vi "FTW-XML-Query-UpdateFirstElementXML.vi"(0 "Parent Element":refnum<k20>, 5 "XPath Query":string, 7 "New XML Element":string, 11 "error in":errorcluster) -> (4 "Parent Element out":refnum<k20>, 6 "Updated?":bool, 15 "error out":errorcluster)   [LabVIEW 2013]
uses:
  ftw-dataflow/Core/src/Error/FTW-ERR-ThrowError.vi
  <resource>/objmgr/DOMUserDefRef.rc
panel:
  # "Inputs"
  # "Outputs"
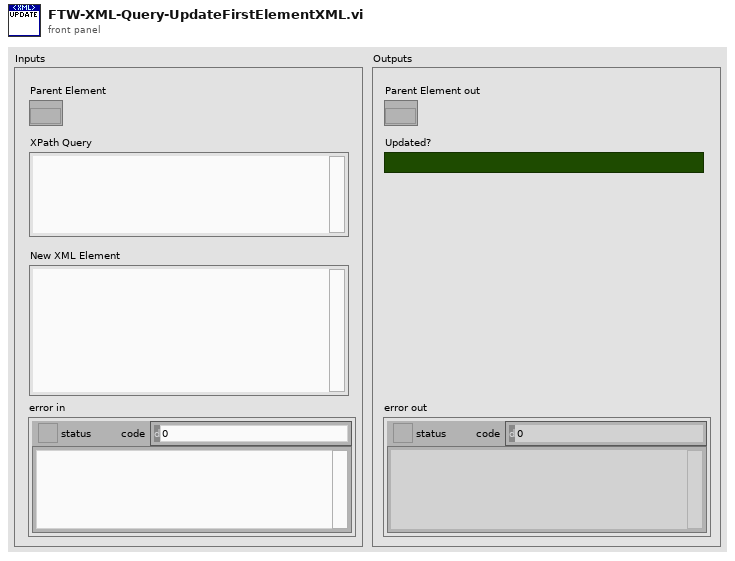
[diagram p1: front panel]
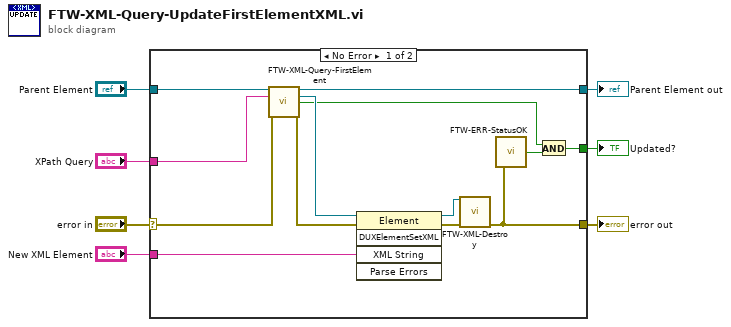
[diagram p0: block diagram]
diagram:
  n1 = case shown="No Error" "error in" {
    selector: "error in" -> [w17 w22]
    tunnel: [w9 w22] -> w7
    tunnel: "Parent Element" -> [w18 w21]
    tunnel: [w16 w21] -> w4
    tunnel: "New XML Element" -> [w20 _]
    tunnel: "XPath Query" -> [w15 _]
    tunnel: [w10 _] -> w1
    frame No Error {
      n2 = call "FTW-XML-Query-FirstElement.vi"("XML Node"=w18, "XPath Query"=w15, "error in"=w17) -> ("XML Node out"=w16:refnum<k20>, "First Matched Element"=w13:refnum<k20>, "Found?"=w11:bool, "error out"=w14:errorcluster)  [unwired: 8 in, 1 out]
      n3 = invoke class="Element" method="DUXElementSetXML"(reference=w13, error in=w14, "XML String"=w20) -> (reference out=w12:refnum<k20>, error out=w19:errorcluster)  [unwired: 2 in, 3 out]
      n4 = call "FTW-XML-Destroy.vi"("XML Node"=w12, "error in"=w19) -> ("error out"=w9:errorcluster)  [unwired: 13 in]
      n5 = call "FTW-ERR-StatusOK.vi"("error to check"=w9) -> ("Status OK?"=w8:bool)
      n6 = And(x=w11, y=w8) -> (x .and. y?=w10:bool)
    }
    frame Error {
    }
  }
  "error out" <- w7
  "Parent Element out" <- w4
  "Updated?" <- w1
